vi "Dac_Output_cam_trig.vi"(0 "File to read":path=path "C:/Users/Hannah/Downloads/newcalibration_voice coil input_25msflyback_3075datapoints.txt", 1 "Image acquisition time (ms)":dbl=1000.0, 2 "Delay between frames":dbl=25.0, 3 "Number of lasers":dbl=3.0, 4 "stop":bool, 5 "error in":errorcluster) -> (19 "error out":errorcluster)   [LabVIEW 2020]
uses:
  <vilib>/DAQmx/write.llb/DAQmx Write (Analog Wfm 1Chan NSamp).vi
  <vilib>/Utility/file.llb/Read Delimited Spreadsheet (DBL).vi
  <vilib>/DAQmx/create/channels.llb/DAQmx Create Channel (CO-Pulse Generation-Ticks).vi
  <vilib>/DAQmx/configure/timing.llb/DAQmx Timing (Implicit).vi
  <vilib>/DAQmx/create/channels.llb/DAQmx Create Channel (AO-Voltage-Basic).vi
  <vilib>/DAQmx/configure/timing.llb/DAQmx Timing (Sample Clock).vi
  <vilib>/DAQmx/miscellaneous.llb/DAQmx Fill In Error Info.vi
  <vilib>/DAQmx/create/channels.llb/DAQmx Create Channel (CO-Pulse Generation-Frequency).vi
  <resource>/objmgr/daqmx.rc
panel:
  out "LabVIEW generated Sawtooth input (blue) and Camera trigger (red)":waveform(dbl)(graph)={"t0"=timestamp(0 s since 1904-01-01), "dt"=1.0, "Y"=array[3075 elements]}
  out "# Samples written per channel":u32=3075
  out "actual frequency":dbl=1000.0
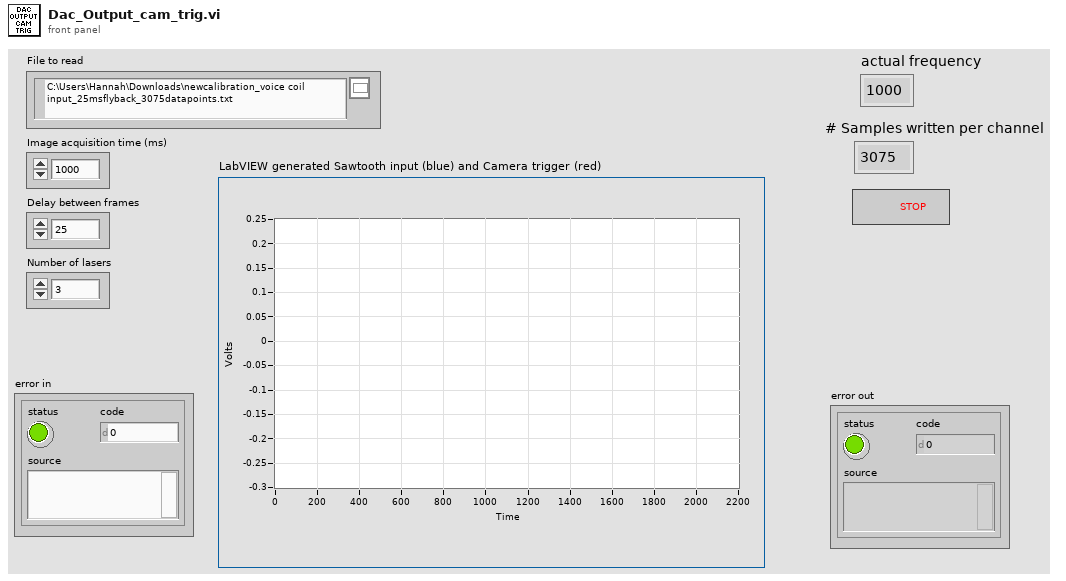
[diagram p1: front panel]
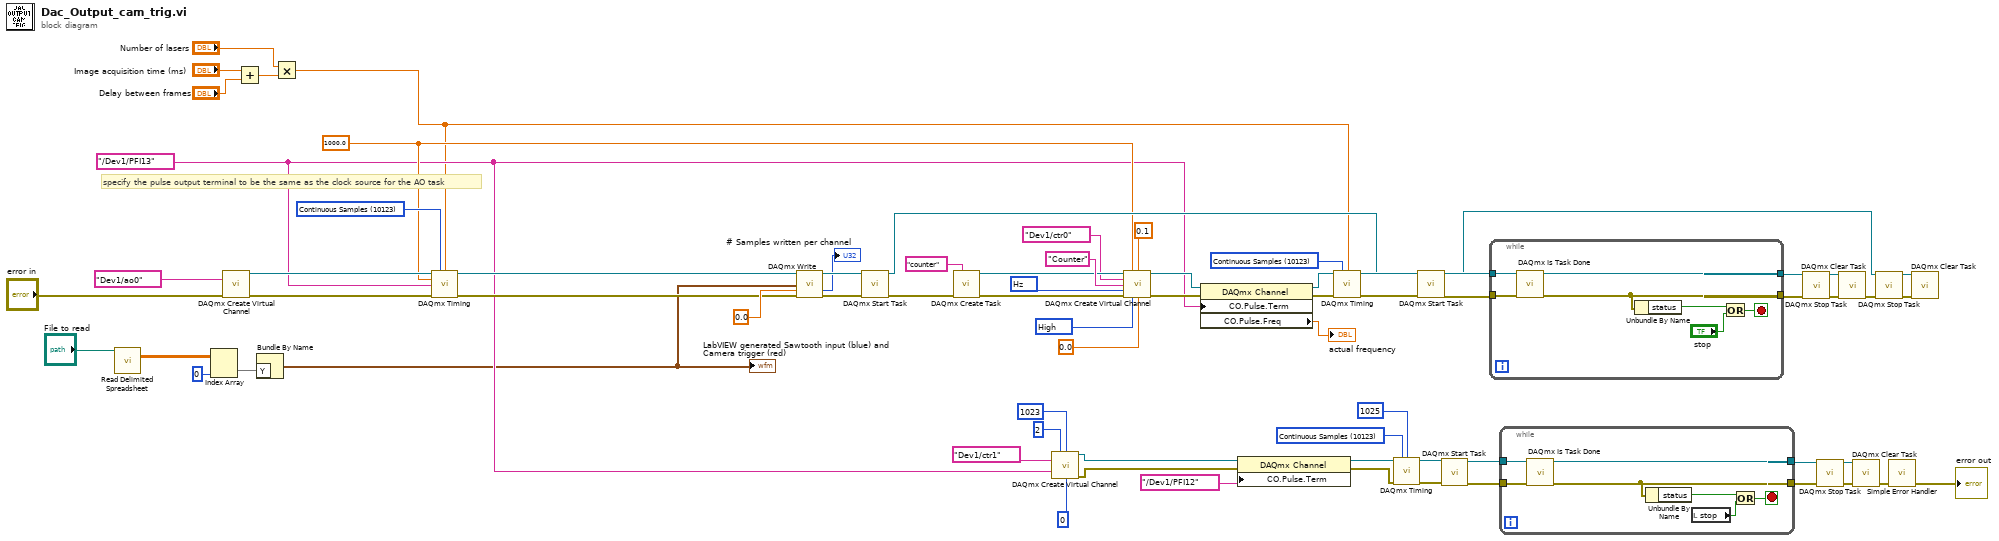
[diagram p0: block diagram]
diagram:
  w18 = 10123 items=["Finite Samples"=10178, "Continuous Samples"=10123, "Hardware Timed Single Point"=12522] ("sample mode")
  w44 = 10192 items=["High"=10192, "Low"=10214] ("idle state")
  w45 = 10373 items=["Hz"=10373] ("units")
  w15 = tag "/Dev1/PFI13" ("CO.Pulse.Term")
  w32 = 10123 items=["Finite Samples"=10178, "Continuous Samples"=10123, "Hardware Timed Single Point"=12522] ("sample mode")
  w28 = 1000.0 ("rate")
  w70 = 10123 items=["Finite Samples"=10178, "Continuous Samples"=10123, "Hardware Timed Single Point"=12522] ("sample mode")
  # "specify the pulse output terminal to be the same as the clock source for the AO task"
  n1 = call-poly <vilib>:"Read Delimited Spreadsheet.vi"("file path (dialog if empty)"="File to read") -> ("all rows"=w13:dbl[][])  [unwired: 9 in, 5 out]
  n2 = Index Array(array=w13, index (col)=0 ("disabled index (col)")) -> (element=w11:dbl[])  [unwired: 1 in]
  n3 = call-poly <vilib>:"DAQmx Create Virtual Channel.vi"("physical channels"=tag "Dev1/ao0", "error in"="error in") -> ("task out"=w72:refnum<k21>, "error out"=w71:errorcluster)  [unwired: 12 in]
  n4 = Add(x="Image acquisition time (ms)", y="Delay between frames") -> (x+y=w5:dbl)
  n5 = Bundle By Name("Y"=w11) -> (w10:waveform(dbl))  [unwired: 1 in]
  "LabVIEW generated Sawtooth input (blue) and Camera trigger (red)" <- w10
  n6 = Multiply(x="Number of lasers", y=w5) -> (x*y=w3:dbl)
  n7 = call-poly <vilib>:"DAQmx Timing.vi"("task/channels in"=w72, "sample mode"=w70, "samples per channel"=w3, "rate"=w28, "source"=w15, "error in"=w71) -> ("task out"=w37:refnum<k21>, "error out"=w36:errorcluster)  [unwired: 8 in]
  n8 = call-poly <vilib>:"DAQmx Write.vi"("task/channels in"=w37, "data"=w10, "timeout"=0.0, "error in"=w36) -> ("task out"=w50:refnum<k21>, "number of samples written per channel"=→"# Samples written per channel":u32, "error out"=w49:errorcluster)  [unwired: 9 in]
  n9 = call <vilib>:"DAQmx Start Task.vi"("task/channels in"=w50, "error in"=w49) -> ("task out"=w43:refnum<k21>, "error out"=w42:errorcluster)  [unwired: 12 in]
  n10 = call <vilib>:"DAQmx Create Task.vi"("new task name"="counter", "error in"=w42) -> ("task out"=w65:refnum<k21>, "error out"=w63:errorcluster)  [unwired: 12 in]
  n11 = call-poly <vilib>:"DAQmx Create Virtual Channel.vi"("high ticks"=u32 2, "low ticks"=u32 1023, "counter"=tag "Dev1/ctr1", "source of ticks"=w15, "initial delay"=u32 0) -> ("task out"=w27:refnum<k21>, "error out"=w26:errorcluster)  [unwired: 9 in]
  n12 = call-poly <vilib>:"DAQmx Create Virtual Channel.vi"("task in"=w65, "frequency"=w28, "duty cycle"=0.1, "counter"=tag "Dev1/ctr0", "name to assign"="Counter", "units"=w45, "error in"=w63, "idle state"=w44, "initial delay"=0.0) -> ("task out"=w62:refnum<k21>, "error out"=w61:errorcluster)  [unwired: 5 in]
  n13 = property class="DAQmx Channel"(reference=w62, error in=w61, "CO.Pulse.Term"=w15) -> (reference out=w58:refnum<k21>, error out=w59:errorcluster, "CO.Pulse.Freq"=→"actual frequency":dbl)
  n14 = property class="DAQmx Channel"(reference=w27, error in=w26, "CO.Pulse.Term"=tag "/Dev1/PFI12") -> (reference out=w20:refnum<k21>, error out=w19:errorcluster)
  n15 = call-poly <vilib>:"DAQmx Timing.vi"("task/channels in"=w58, "sample mode"=w32, "samples per channel"=w3, "error in"=w59) -> ("task out"=w68:refnum<k21>, "error out"=w67:errorcluster)  [unwired: 10 in]
  n16 = call-poly <vilib>:"DAQmx Timing.vi"("task/channels in"=w20, "sample mode"=w18, "samples per channel"=1025, "error in"=w19) -> ("task out"=w17:refnum<k21>, "error out"=w16:errorcluster)  [unwired: 10 in]
  n17 = call <vilib>:"DAQmx Start Task.vi"("task/channels in"=w68, "error in"=w67) -> ("task out"=w39:refnum<k21>, "error out"=w51:errorcluster)  [unwired: 12 in]
  n18 = call <vilib>:"DAQmx Start Task.vi"("task/channels in"=w17, "error in"=w16) -> ("task out"=w24:refnum<k21>, "error out"=w23:errorcluster)  [unwired: 12 in]
  n19 = while {
    tunnel: w43 -> [w79]
    tunnel: w51 -> [w78]
    tunnel: [w77] -> w54
    tunnel: [w76] -> w55
    stop <- w73 stop-if-true
    n20 = call <vilib>:"DAQmx Is Task Done.vi"("task/channels in"=w79, "error in"=w78) -> ("task out"=w77:refnum<k21>, "error out"=w76:errorcluster)  [unwired: 11 in, 1 out]
    n21 = Unbundle By Name(w76) -> ("status"=w75:bool)
    n22 = Or(x=w75, y="stop") -> (x .or. y?=w73:bool)
  }
  n23 = while {
    tunnel: w24 -> [w86]
    tunnel: w23 -> [w85]
    tunnel: [w84] -> w22
    tunnel: [w83] -> w21
    stop <- w81 stop-if-true
    n24 = call <vilib>:"DAQmx Is Task Done.vi"("task/channels in"=w86, "error in"=w85) -> ("task out"=w84:refnum<k21>, "error out"=w83:errorcluster)  [unwired: 11 in, 1 out]
    n25 = Unbundle By Name(w83) -> ("status"=w82:bool)
    n26 = local read "stop"() -> (w80:bool)
    n27 = Or(x=w82, y=w80) -> (x .or. y?=w81:bool)
  }
  n28 = call <vilib>:"DAQmx Stop Task.vi"("task/channels in"=w54, "error in"=w55) -> ("task out"=w53:refnum<k21>, "error out"=w52:errorcluster)  [unwired: 12 in]
  n29 = call <vilib>:"DAQmx Stop Task.vi"("task/channels in"=w22, "error in"=w21) -> ("task out"=w30:refnum<k21>, "error out"=w31:errorcluster)  [unwired: 12 in]
  n30 = call <vilib>:"DAQmx Clear Task.vi"("task in"=w53, "error in"=w52) -> ("error out"=w38:errorcluster)  [unwired: 13 in]
  n31 = call <vilib>:"DAQmx Clear Task.vi"("task in"=w30, "error in"=w31) -> ("error out"=w29:errorcluster)  [unwired: 13 in]
  n32 = call <vilib>:"DAQmx Stop Task.vi"("task/channels in"=w39, "error in"=w38) -> ("task out"=w56:refnum<k21>, "error out"=w57:errorcluster)  [unwired: 12 in]
  n33 = call <vilib>:"Simple Error Handler.vi"("error in (no error)"=w29) -> ("error out"=→"error out":errorcluster)  [unwired: 4 in, 4 out]
  n34 = call <vilib>:"DAQmx Clear Task.vi"("task in"=w56, "error in"=w57) -> ()  [unwired: 13 in, 1 out]
